vi "Laser Pos Judge.vi"(5 "Allowed area L_green":T2={"Left"=0, "Top"=0, "Right"=624, "Bottom"=2160}, 7 "Allowed area R_green":T2={"Left"=1936, "Top"=0, "Right"=2560, "Bottom"=2160}, 8 "error in (no error)":errorcluster, 10 "Difference between points":i32=30, 11 "Refnum in":T1) -> (0 "error out":errorcluster, 1 "Boolean":bool, 2 "Absolute R-L Score":i32, 3 "Refnum out":T1)   [LabVIEW 2019, in "Image.lvlib"]
uses:
  <vilib>/vision/Image Controls.llb/IMAQ Image.ctl
  Image.lvlib
panel:
  out "L":i32
  out "R":i32
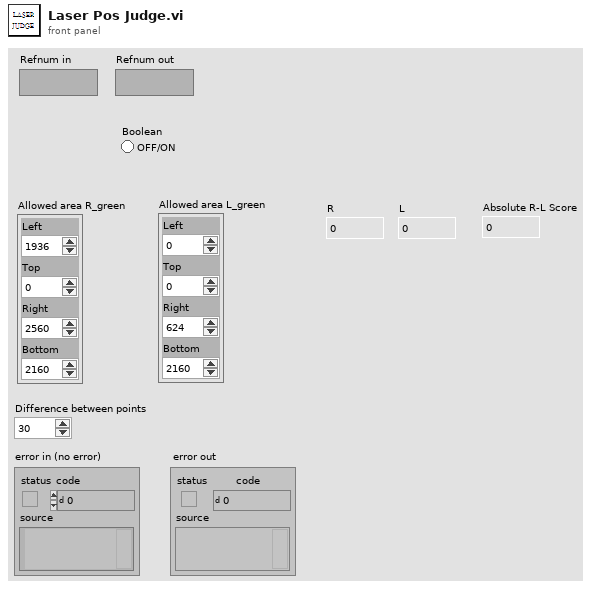
[diagram p1: front panel]
types:
  T1 = typedef "IMAQ Image.ctl" = refnum<image>
  T2 = cluster{"Left":i32, "Top":i32, "Right":i32, "Bottom":i32}
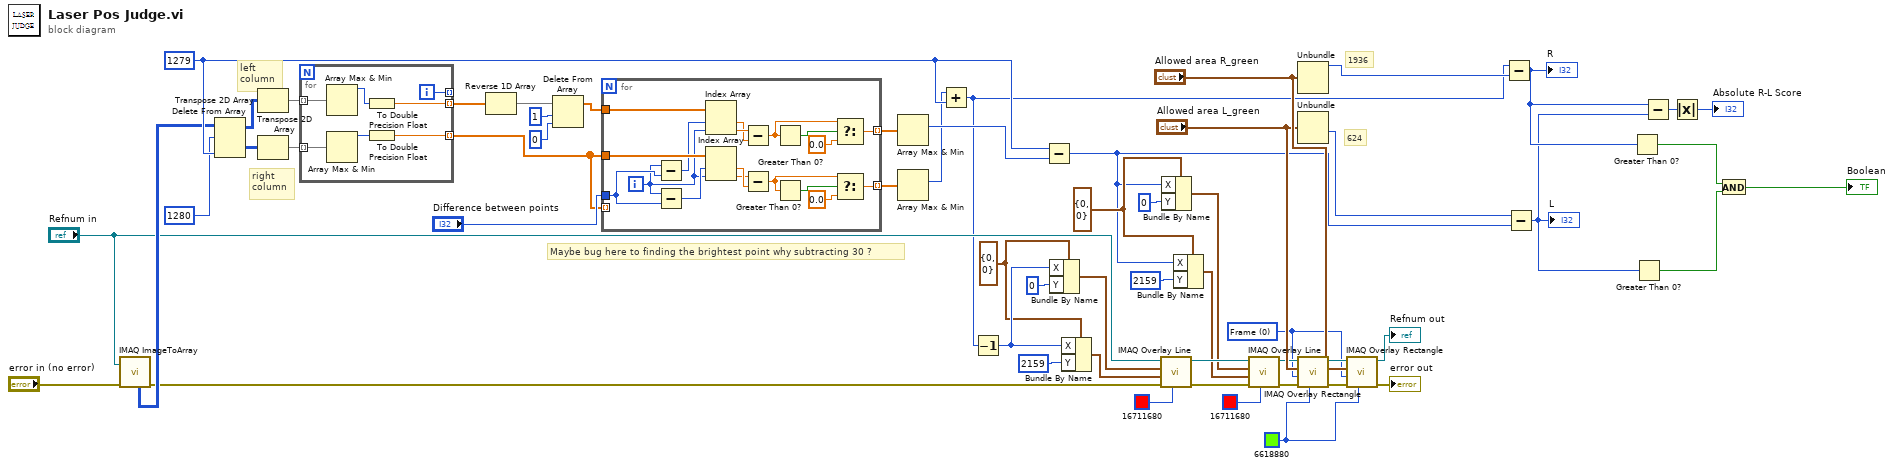
[diagram p0: block diagram]
diagram:
  w39 = cluster{"X":i32, "Y":i32} {"X"=0, "Y"=0} ("Start Point")
  w48 = u32 0 items=["Frame", "Fill", "Highlight"] ("Drawing Mode (Frame)")
  w49 = u32 6618880 ("Color")
  w25 = cluster{"X":i32, "Y":i32} {"X"=0, "Y"=0} ("Start Point")
  w46 = 1279 ("disabled index (col)")
  # "Maybe bug here to finding the brightest point why subtracting 30 ?"
  # "624"
  # "1936"
  # "left \ncolumn"
  # "right\ncolumn"
  n1 = call "IMAQ ImageToArray"("error in (no error)"="error in (no error)", "Image"="Refnum in") -> ("Image Pixels (U16)"=w19:u16[][], "error out"=w12:errorcluster)  [unwired: 2 in, 3 out]
  n2 = Delete From Array(array=w19, length=1280, index (col)=w46) -> (deleted portion=w21:u16[][], array with subset deleted=w34:u16[][])  [unwired: 1 in]
  n3 = Transpose 2D Array(2D array=w34) -> (transposed array=w54:u16[][])
  n4 = Transpose 2D Array(2D array=w21) -> (transposed array=w22:u16[][])
  n5 = for {
    tunnel: w22 -> [w63] mode=indexing
    tunnel: [w61] -> w23 mode=indexing
    tunnel: [w64] -> _ mode=indexing
    tunnel: w54 -> [w59] mode=indexing
    tunnel: [w58] -> w55 mode=indexing
    i -> [w64]
    n6 = Array Max & Min(array=w59) -> (max value=w60:u16)  [unwired: 3 out]
    n7 = Array Max & Min(array=w63) -> (max value=w62:u16)  [unwired: 3 out]
    n8 = To Double Precision Float(number=w60) -> (double precision float=w58:dbl)
    n9 = To Double Precision Float(number=w62) -> (double precision float=w61:dbl)
  }
  n10 = Reverse 1D Array(array=w55) -> (reversed array=w45:dbl[])
  n11 = Delete From Array(array=w45, length=1, index=0) -> (array with subset deleted=w56:dbl[])  [unwired: 1 out]
  n12 = for {
    tunnel: w23 -> [_] mode=indexing
    tunnel: w23 -> [w82]
    tunnel: [w75] -> w24 mode=indexing
    tunnel: "Difference between points" -> [w69]
    tunnel: w56 -> [w65]
    tunnel: [w70] -> w57 mode=indexing
    i -> [w68]
    n13 = Subtract(x=w68, y=w69) -> (x-y=w71:i32)
    n14 = Subtract(x=w68, y=w69) -> (x-y=w81:i32)
    n15 = Index Array(array=w65, index #1=w71, index #2=w68) -> (element #1=w66:dbl, element #2=w67:dbl)
    n16 = Index Array(array=w82, index #1=w81, index #2=w68) -> (element #1=w80:dbl, element #2=w79:dbl)
    n17 = Subtract(x=w67, y=w66) -> (x-y=w74:dbl)
    n18 = Subtract(x=w79, y=w80) -> (x-y=w76:dbl)
    n19 = Greater Than 0?(x=w74) -> (x > 0?=w73:bool)
    n20 = Greater Than 0?(x=w76) -> (x > 0?=w77:bool)
    n21 = Select(t=w74, s=w73, f=0.0) -> (s? t:f=w70:dbl)
    n22 = Select(t=w76, s=w77, f=0.0) -> (s? t:f=w75:dbl)
  }
  n23 = Array Max & Min(array=w57) -> (max index (indices)=w47:i32)  [unwired: 3 out]
  n24 = Array Max & Min(array=w24) -> (max index (indices)=w31:i32)  [unwired: 3 out]
  n25 = Add(x=w31, y=w46) -> (x+y=w10:i32)
  n26 = Decrement(x=w10) -> (x-1=w42:i32)
  n27 = Subtract(x=w46, y=w47) -> (x-y=w8:i32)
  n28 = Bundle By Name(cluster=w25, "X"=w42, "Y"=0) -> (w26:cluster{"X":i32, "Y":i32})
  n29 = Bundle By Name(cluster=w25, "X"=w42, "Y"=2159) -> (w27:cluster{"X":i32, "Y":i32})
  n30 = call "IMAQ Overlay Line"("Color"=u32 16711680, "error in (no error)"=w12, "End Point"=w27, "Start Point"=w26, "Image"="Refnum in") -> ("error out"=w17:errorcluster, "Image Out"=w41:T1)  [unwired: 5 in]
  n31 = Bundle By Name(cluster=w39, "X"=w8, "Y"=0) -> (w38:cluster{"X":i32, "Y":i32})
  n32 = Bundle By Name(cluster=w39, "X"=w8, "Y"=2159) -> (w40:cluster{"X":i32, "Y":i32})
  n33 = call "IMAQ Overlay Line"("Color"=u32 16711680, "error in (no error)"=w17, "End Point"=w40, "Start Point"=w38, "Image"=w41) -> ("error out"=w16:errorcluster, "Image Out"=w51:T1)  [unwired: 5 in]
  n34 = Unbundle("Allowed area R_green") -> ("Left"=w11:i32)  [unwired: 3 out]
  n35 = Unbundle("Allowed area L_green") -> ("Right"=w9:i32)  [unwired: 3 out]
  n36 = call "IMAQ Overlay Rectangle"("Color"=w49, "error in (no error)"=w16, "Drawing Mode (Frame)"=w48, "Rectangle"="Allowed area L_green", "Image"=w51) -> ("error out"=w15:errorcluster, "Image Out"=w50:T1)  [unwired: 5 in]
  n37 = call "IMAQ Overlay Rectangle"("Color"=w49, "error in (no error)"=w15, "Drawing Mode (Frame)"=w48, "Rectangle"="Allowed area R_green", "Image"=w50) -> ("error out"=→"error out":errorcluster, "Image Out"=→"Refnum out":T1)  [unwired: 5 in]
  n38 = Subtract(x=w10, y=w11) -> (x-y=w4:i32)
  "R" <- w4
  n39 = Subtract(x=w9, y=w8) -> (x-y=w3:i32)
  "L" <- w3
  n40 = Greater Than 0?(x=w4) -> (x > 0?=w7:bool)
  n41 = Greater Than 0?(x=w3) -> (x > 0?=w6:bool)
  n42 = Subtract(x=w4, y=w3) -> (x-y=w2:i32)
  n43 = Absolute Value(x=w2) -> (abs(x)=→"Absolute R-L Score":i32)
  n44 = And(x=w7, y=w6) -> (x .and. y?=→"Boolean":bool)
